vi "PC_CallRTMultipleVIsGuidedMunitions.vi"(8 "error in (no error)":errorcluster, 11 "StepParameter":T2[](array[typedef])) -> (0 "error out":errorcluster, 3 "StepOutputParameter":T1[](array[typedef]))   [LabVIEW 2010]
uses:
  Ctls/PC_DynCallVIParameter.ctl
  Ctls/PC_DynCallVIOutputParameter.ctl
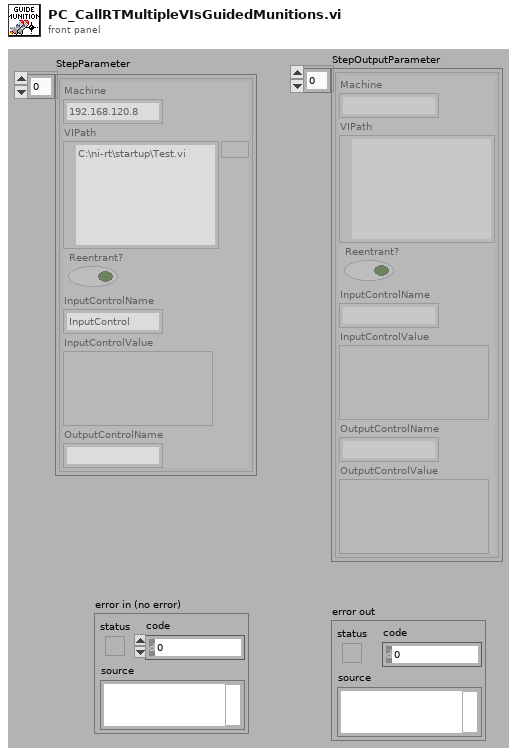
[diagram p1: front panel]
types:
  T1 = typedef "PC_DynCallVIOutputParameter.ctl" = cluster{"Machine":string, "VIPath":path, "Reentrant?":bool, "InputControlName":string, "InputControlValue":variant, "OutputControlName":string, "OutputControlValue":variant}
  T2 = typedef "PC_DynCallVIParameter.ctl" = cluster{"Machine":string, "VIPath":path, "Reentrant?":bool, "InputControlName":string, "InputControlValue":variant, "OutputControlName":string}
  T3 = enum32{"Bad", "Idle", "Run top level", "Running"}
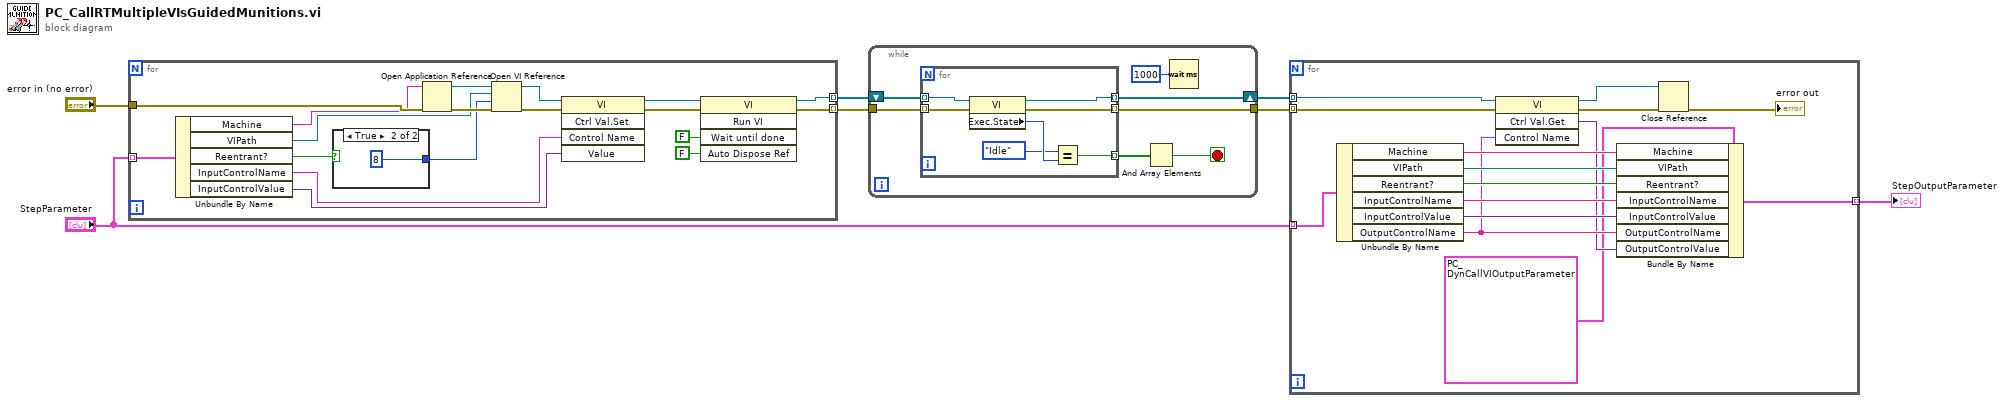
[diagram p0: block diagram]
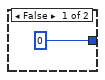
[diagram p2: hidden frame]
diagram:
  n1 = for {
    tunnel: "error in (no error)" -> [w17]
    tunnel: [w16] -> w6 mode=indexing
    tunnel: [w15] -> w5 mode=indexing
    tunnel: "StepParameter" -> [w14] mode=indexing
    n2 = Unbundle By Name(w14) -> ("Machine"=w13:string, "VIPath"=w12:path, "Reentrant?"=w11:bool, "InputControlName"=w10:string, "InputControlValue"=w9:variant)
    n3 = case shown="True" w11 {
      tunnel: [0 ("options") 8 ("options")] -> w21
      frame False {
      }
      frame True {
      }
    }
    n4 = Open Application Reference(8:w17, 11:w13) -> (0:w24:errorcluster, 3:w25:refnum<vi>)  [unwired: 2 in]
    n5 = Open VI Reference(application reference (local)=w25, vi path=w12, options=w21, error in (no error)=w24) -> (vi reference=w20:refnum<vi>, error out=w19:errorcluster)  [unwired: 2 in]
    n6 = invoke class="VI" method="Ctrl Val.Set"(reference=w20, error in=w19, "Control Name"=w10, "Value"=w9) -> (reference out=w8:refnum<vi>, error out=w18:errorcluster)  [unwired: 1 in, 3 out]
    n7 = invoke class="VI" method="Run VI"(reference=w8, error in=w18, "Wait until done"=FALSE ("Wait Until Done"), "Auto Dispose Ref"=FALSE ("Auto Dispose Reference")) -> (reference out=w16:refnum<vi>, error out=w15:errorcluster)  [unwired: 1 in, 3 out]
  }
  n8 = while {
    tunnel: w5 -> [w33]
    tunnel: [w31] -> w3
    shift-right: [w32] -> w4
    shift-left: w6 -> [w34]
    stop <- w29 stop-if-true
    n9 = for {
      tunnel: w34 -> [w35] mode=indexing
      tunnel: w33 -> [w41] mode=indexing
      tunnel: [w39] -> w32 mode=indexing
      tunnel: [w38] -> w31 mode=indexing
      tunnel: [w36] -> w30 mode=indexing
      n10 = property class="VI"(reference=w35, error in=w41) -> (reference out=w39:refnum<vi>, error out=w38:errorcluster, "Exec.State"=w40:T3)
      n11 = Equal?(x=T3."Idle", y=w40) -> (x = y?=w36:bool)
    }
    n12 = And Array Elements(Boolean array=w30) -> (logical AND=w29:bool)
    n13 = Wait (ms)(milliseconds to wait=u32 1000) -> ()  [unwired: 1 out]
  }
  n14 = for {
    tunnel: w4 -> [w53] mode=indexing
    tunnel: w3 -> [w52] mode=indexing
    tunnel: "StepParameter" -> [w51] mode=indexing
    tunnel: [w43] -> w1 mode=indexing
    n15 = Unbundle By Name(w51) -> ("Machine"=w50:string, "VIPath"=w49:path, "Reentrant?"=w48:bool, "InputControlName"=w47:string, "InputControlValue"=w46:variant, "OutputControlName"=w45:string)
    n16 = invoke class="VI" method="Ctrl Val.Get"(reference=w53, error in=w52, "Control Name"=w45) -> (reference out=w55:refnum<vi>, error out=w56:errorcluster, "Get Control Value Variant"=w44:variant)  [unwired: 1 in, 1 out]
    n17 = Bundle By Name(cluster=T1 {"Machine"="192.168.120.8", "VIPath"=path "C:/ni-rt/startup/Test.vi", "Reentrant?"=FALSE, "InputControlName"="InputControl", "InputControlValue"=variant, "OutputControlName"="", "OutputControlValue"=variant} ("VIParameter"), "Machine"=w50, "VIPath"=w49, "Reentrant?"=w48, "InputControlName"=w47, "InputControlValue"=w46, "OutputControlName"=w45, "OutputControlValue"=w44) -> (w43:T1)
    n18 = Close Reference(reference=w55, error in (no error)=w56) -> (error out=→"error out":errorcluster)
  }
  "StepOutputParameter" <- w1
